vi "SQLite Insert Calibration Value.vi"(7 "Main":string="0", 8 "error in (no error)":errorcluster, 9 "Calibration Value":T1, 11 "VariableName":string) -> (0 "error out":errorcluster)   [LabVIEW 2017, in "SQLite.lvclass"]
doc: "保存校准数据到DB。在保存之前先调用删除原先校准数据模块。\n2015-11-03 15:56:09\n蒋松\njiangsong@outlook.com"
uses:
  SQLite.lvclass
  Calibration Value.ctl
  SQLiteFileName.ctl
  TabelFullName.ctl
  Calibration Kb and Volt.ctl
  Calibration K and b Array.ctl
  Calibration K and b.ctl
  <vilib>/Utility/error.llb/Trim Whitespace.vi
  <userlib>/sushu/sushu.lvlib
  <userlib>/LabSQL/LabSQL.lvlib
panel:
  out "Insert DB String":string
  in  "error in (no error) 2":errorcluster
  in  "OK":bool
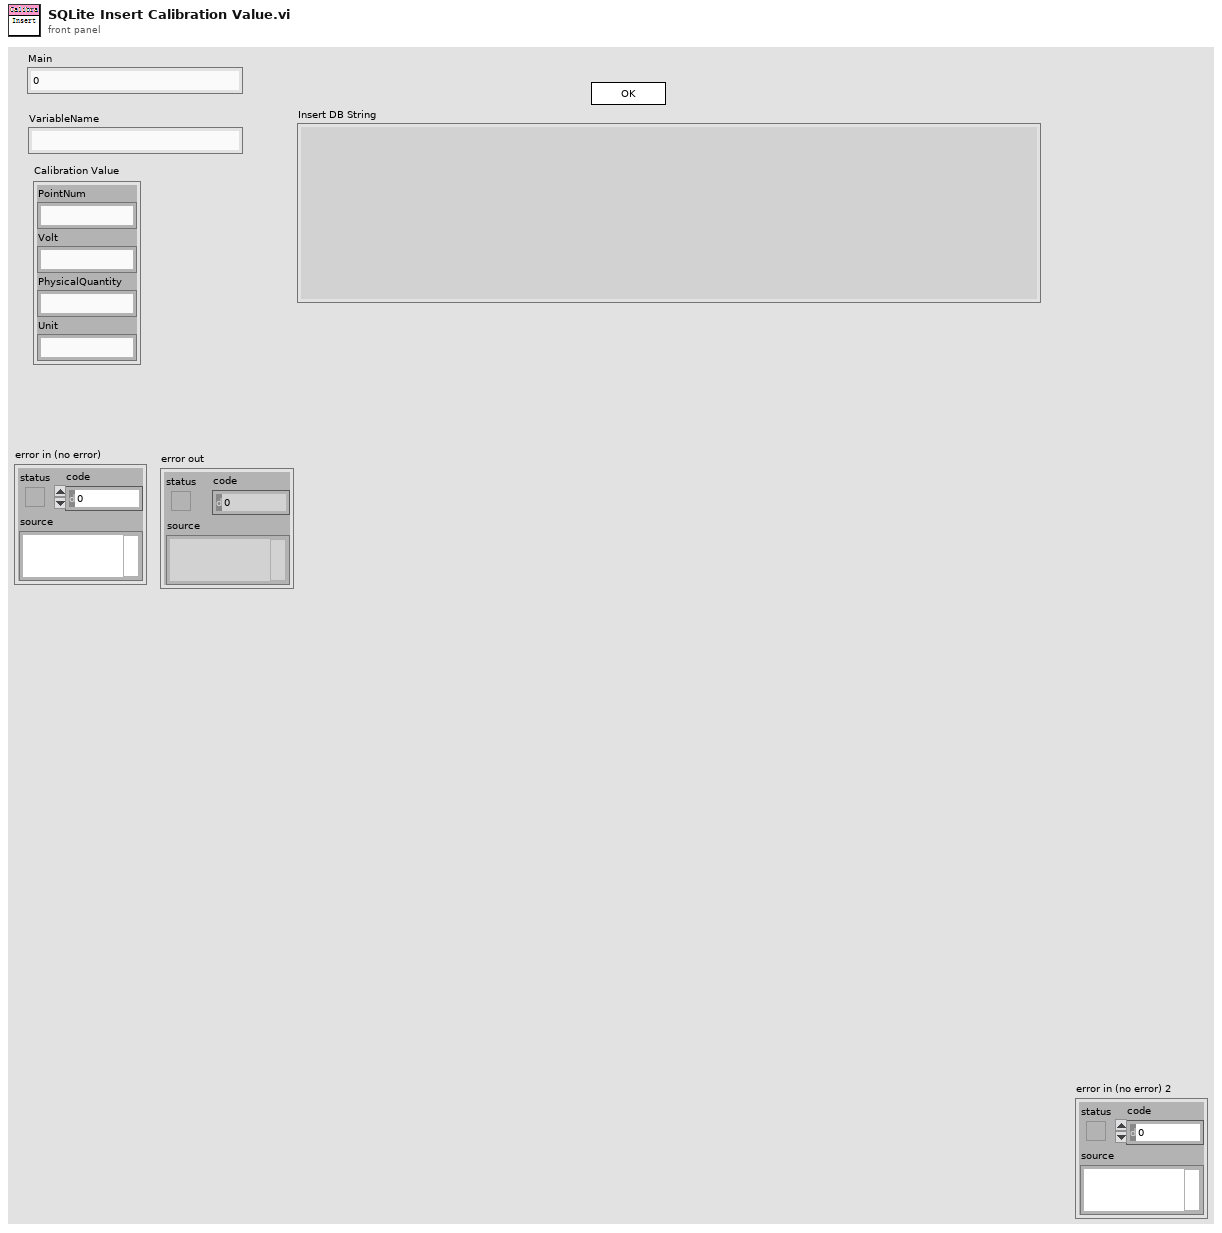
[diagram p1: front panel]
types:
  T1 = typedef "SQLite.lvclass/Calibration Value.ctl" = cluster{"PointNum":string, "Volt":string, "PhysicalQuantity":string, "Unit":string}
  T2 = typedef "SQLite.lvclass/Calibration Kb and Volt.ctl" = cluster{"Kb":T3, "Relation":dbl[][]}
  T3 = typedef "SQLite.lvclass/Calibration K and b Array.ctl" = T4[]
  T4 = typedef "SQLite.lvclass/Calibration K and b.ctl" = cluster{"K":dbl, "b":dbl}
  T5 = typedef "SQLite.lvclass/TabelFullName.ctl" = string
  T6 = typedef "SQLite.lvclass/SQLiteFileName.ctl" = string
  T7 = cluster{"Current VI Reference":refnum<vi>, "Close Panel on Exit?":bool}
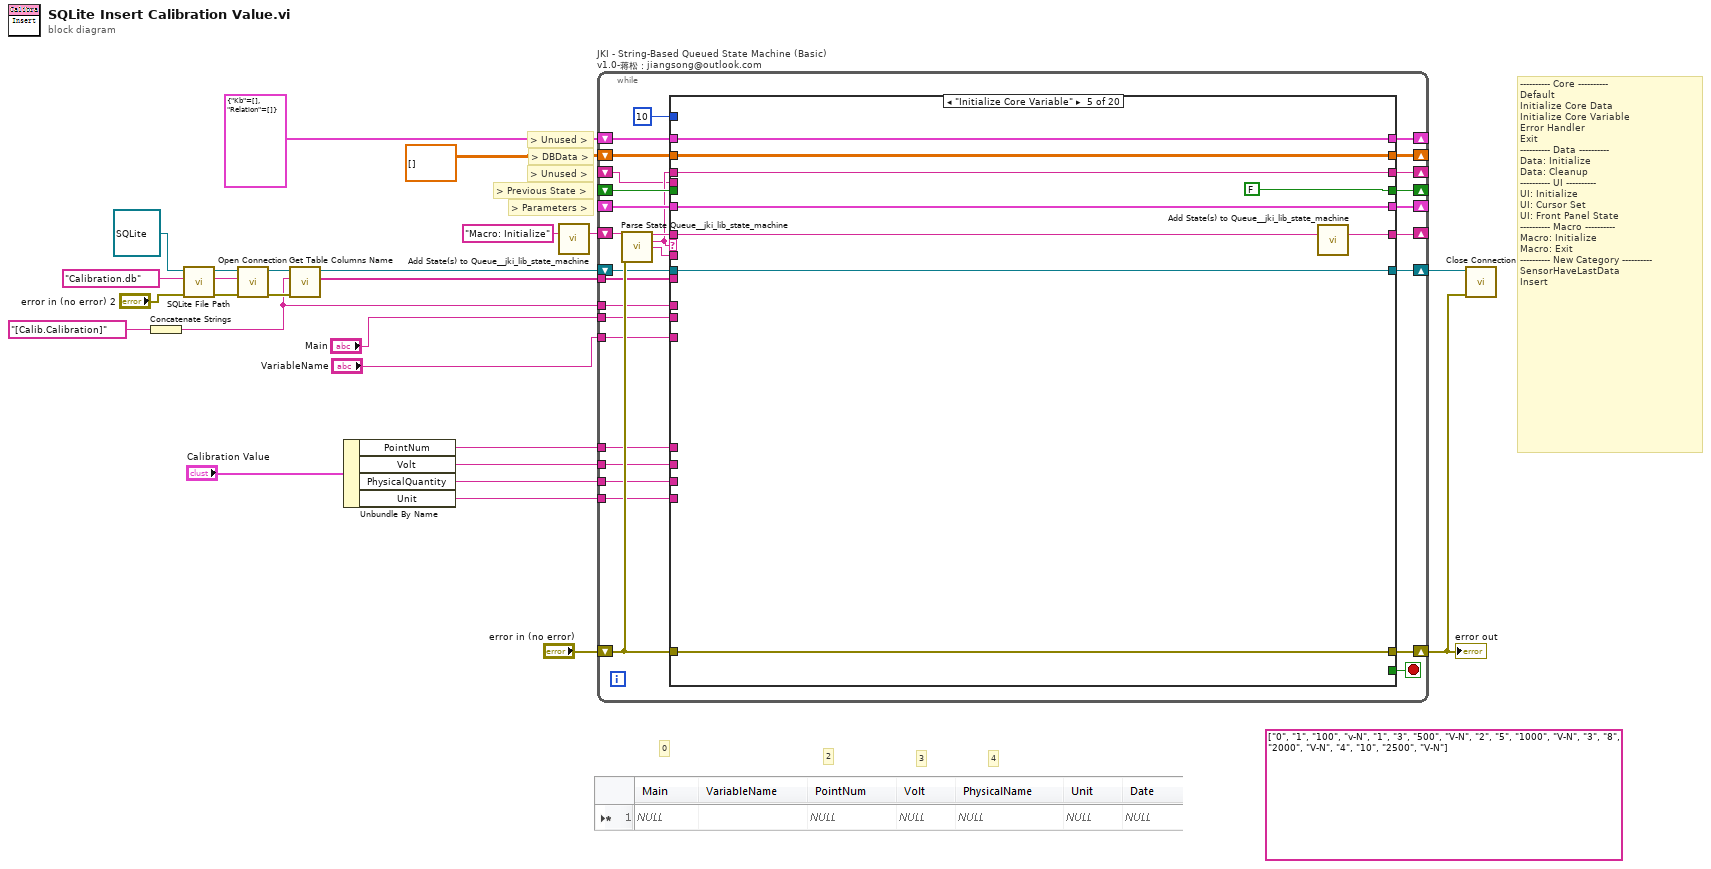
[diagram p0: block diagram]
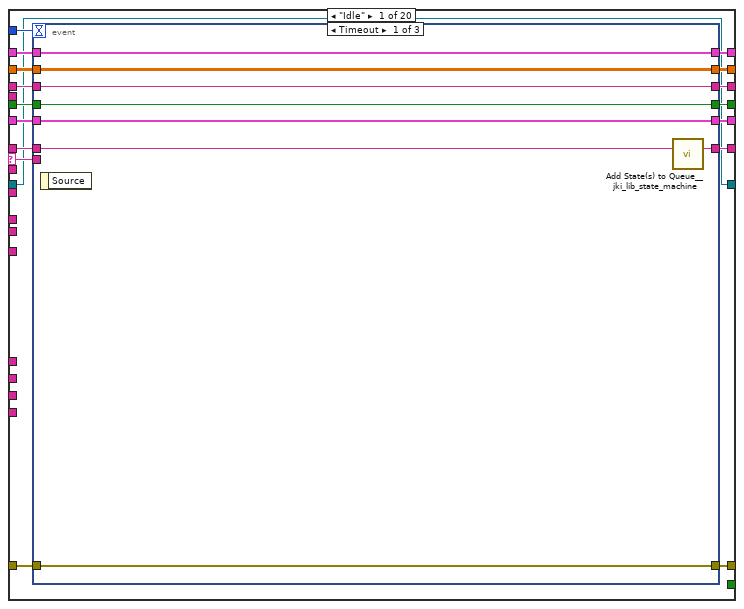
[diagram p2: hidden frame]
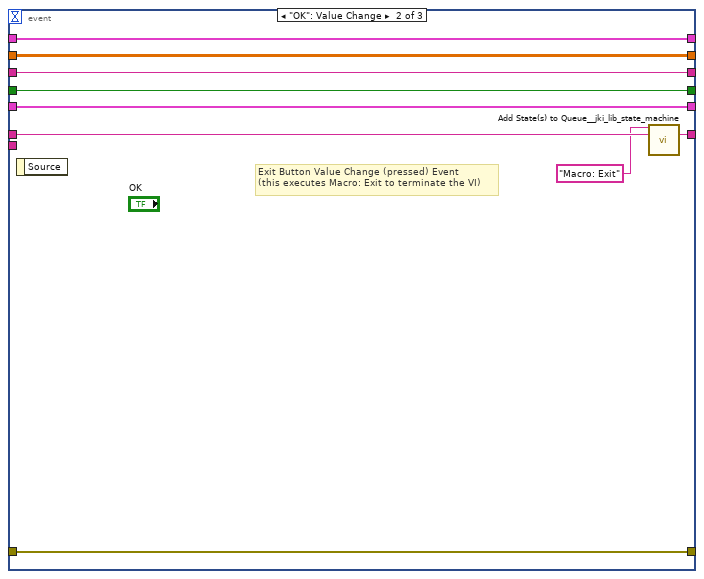
[diagram p3: hidden frame]
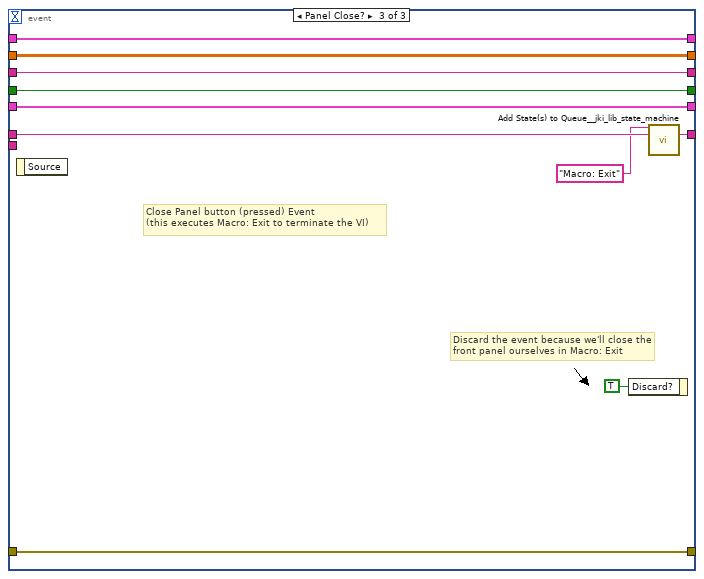
[diagram p4: hidden frame]
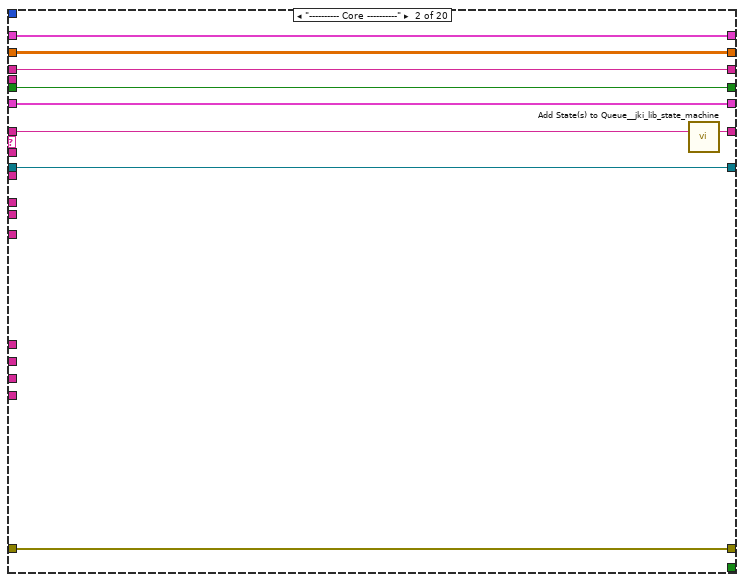
[diagram p5: hidden frame]
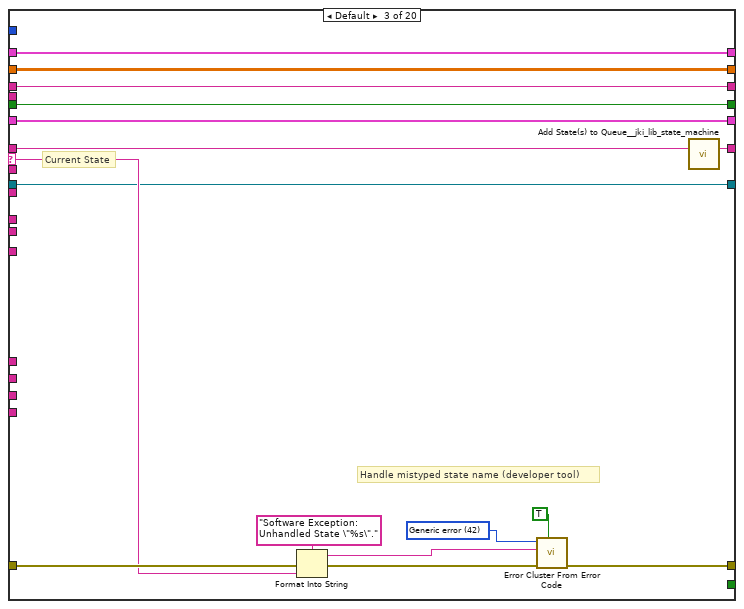
[diagram p6: hidden frame]
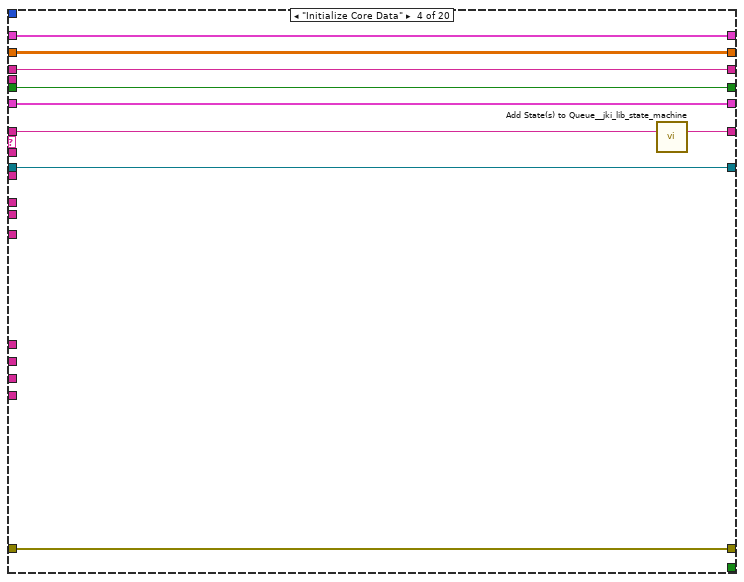
[diagram p7: hidden frame]
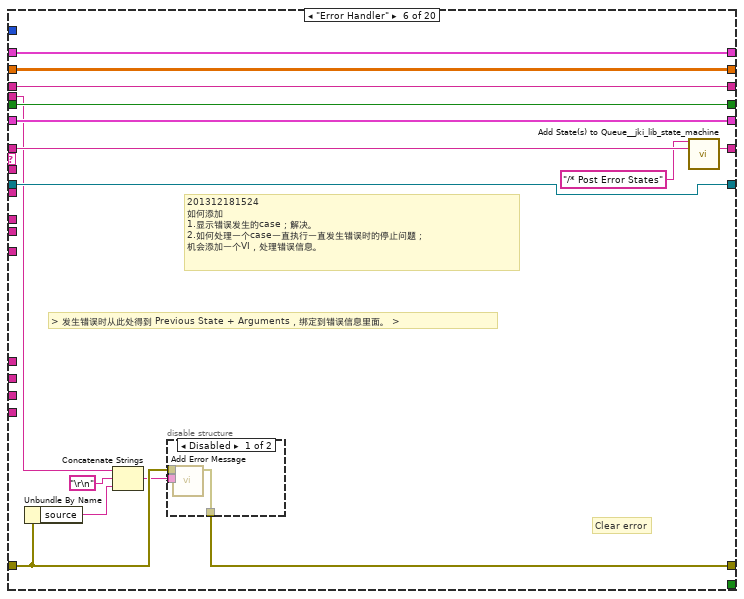
[diagram p8: hidden frame]
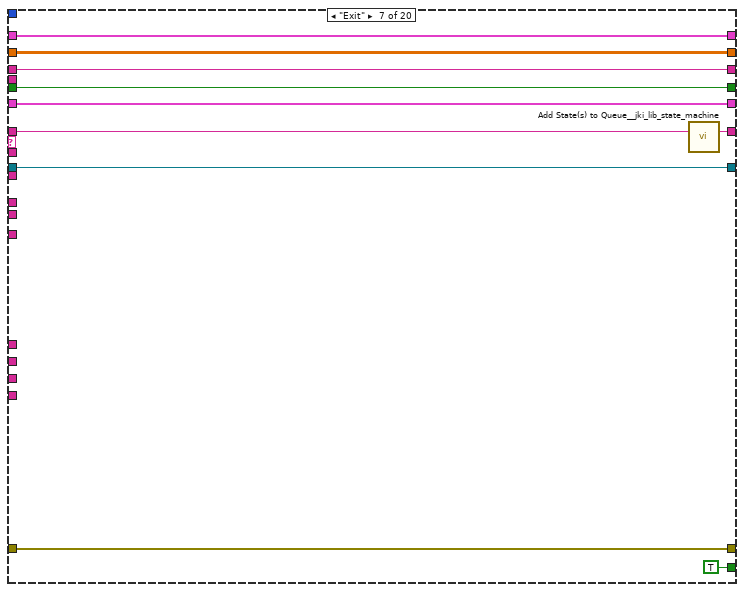
[diagram p10: hidden frame]
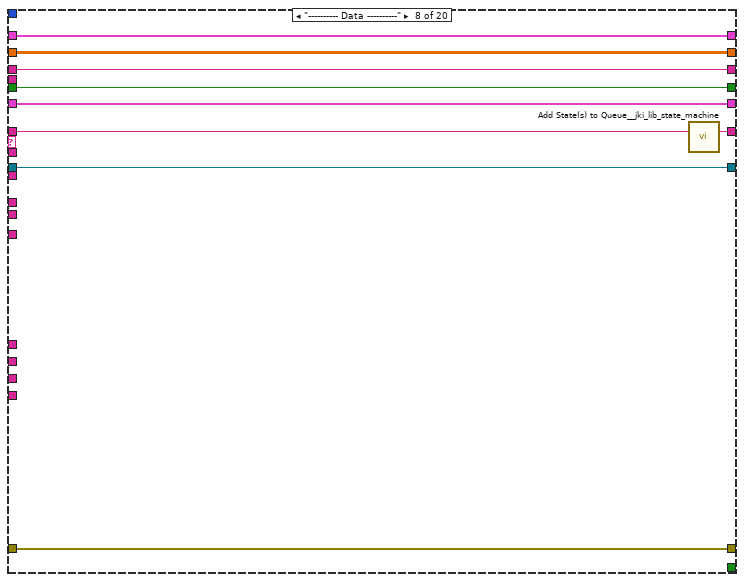
[diagram p11: hidden frame]
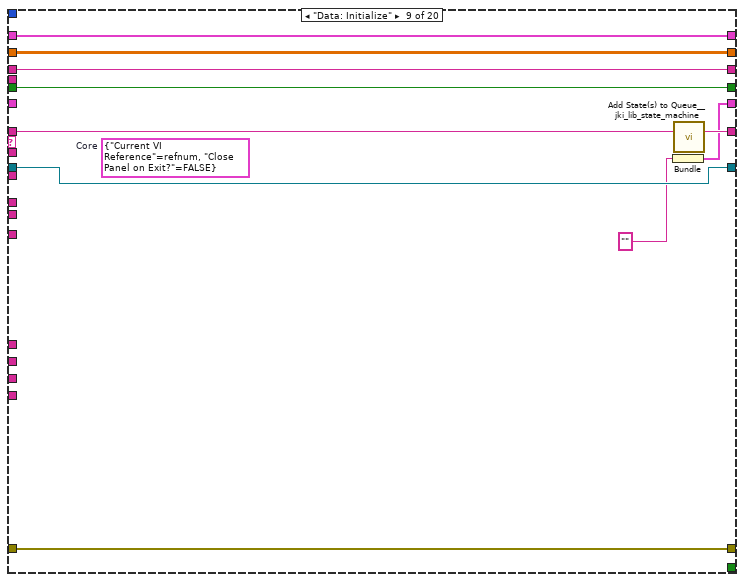
[diagram p12: hidden frame]
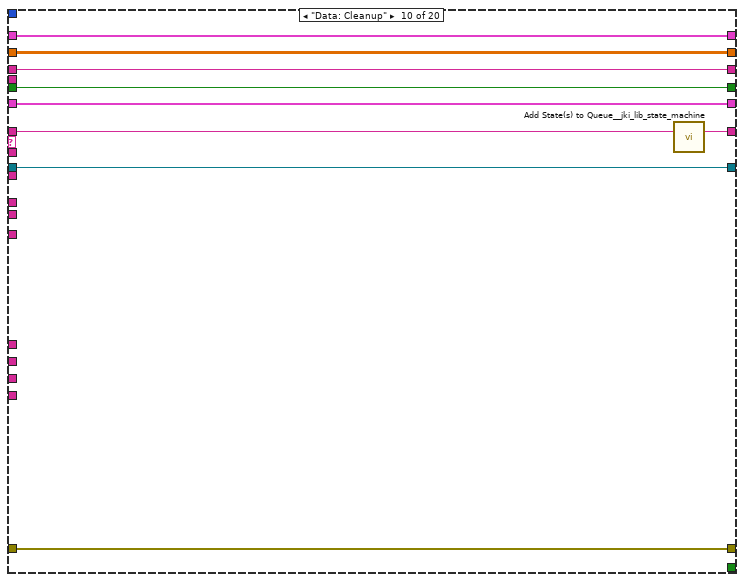
[diagram p13: hidden frame]
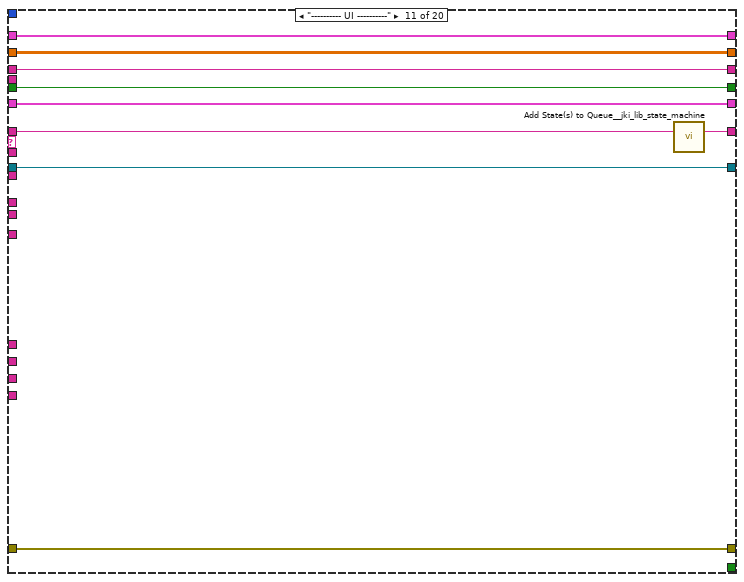
[diagram p14: hidden frame]
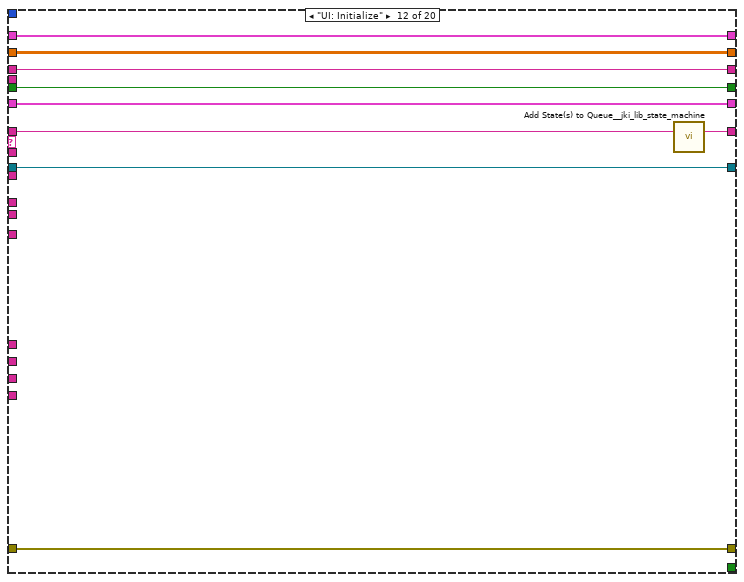
[diagram p15: hidden frame]
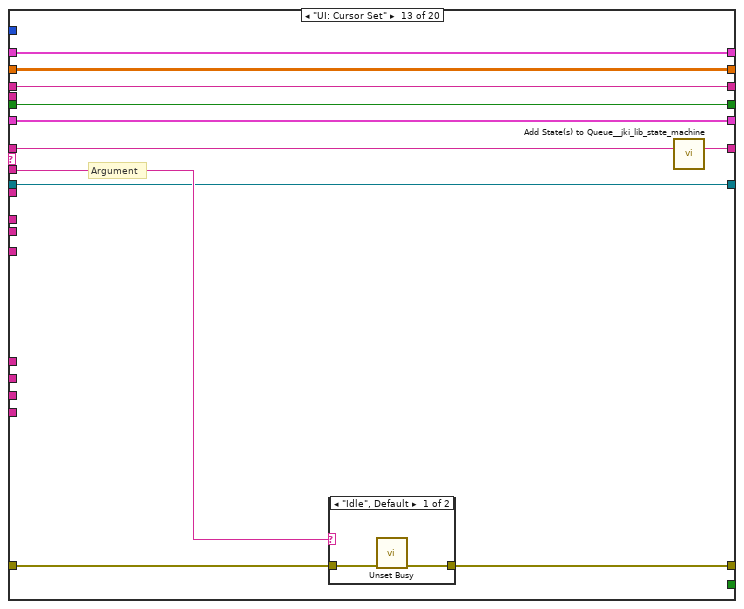
[diagram p16: hidden frame]
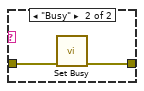
[diagram p17: hidden frame]
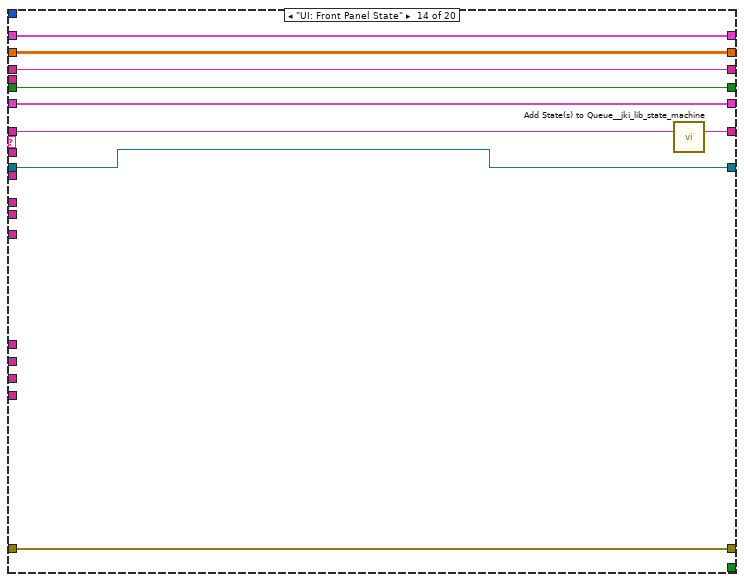
[diagram p18: hidden frame]
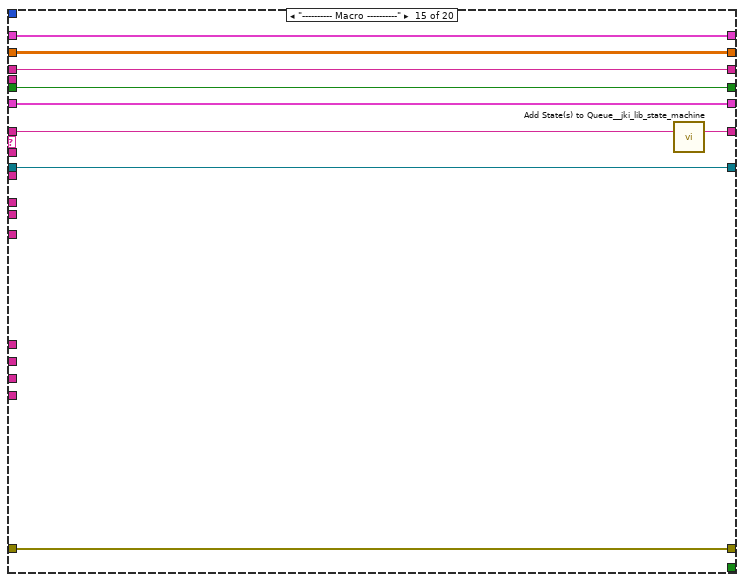
[diagram p19: hidden frame]
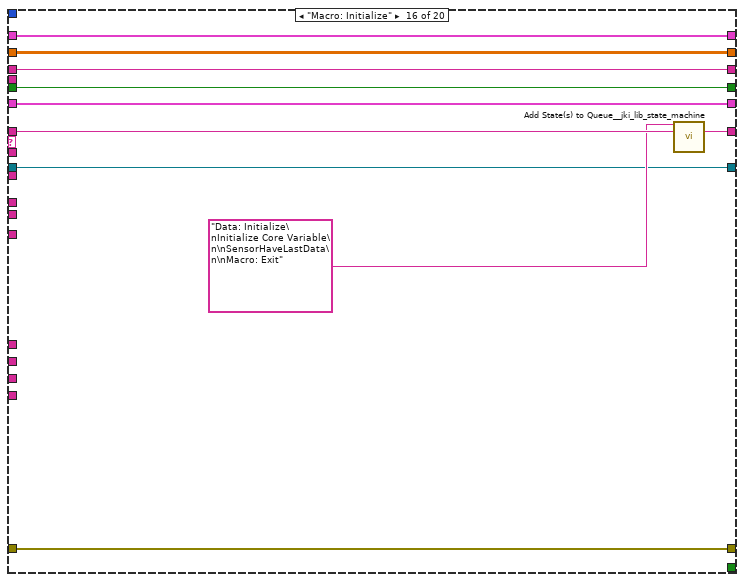
[diagram p20: hidden frame]
diagram:
  (unwired) string[][] [["0", "1", "100", "v-N"], ["1", "3", "500", "V-N"], ["2", "5", "1000", "V-N"], ["3", "8", "2000", "V-N"], ["4", "10", "2500", "V-N"]] ("Result Set 2")
  # "3"
  # "0"
  # "> Parameters >"
  # "> Previous State >"
  # "> Unused >"
  # "> DBData >"
  # "> Unused >"
  # "---------- Core ----------\nDefault\nInitialize Core Data\nInitialize Core Variable\nError Handler\nExit\n---------- Data ----------\nData: Initialize\nData: Cleanup\n---------- UI ----------\nUI: Initialize\nUI: Cursor Set\nUI: Front Panel State\n---------- Macro ----------\nMacro: Initialize\nMacro: Exit\n---------- New Category ----------\nSensorHaveLastData\nInsert"
  # "2"
  # "4"
  n1 = Concatenate Strings(T5 "[Calib.Calibration]" ("TabelFullName")) -> (w9:string)
  n2 = call "SQLite File Path.vi"("error in (no error)"="error in (no error) 2", "SQLiteFileName"=T6 "Calibration.db", "SQLite in"=refnum<class "SQLite.lvclass"> refnum ("SQLite.lvclass")) -> ("error out"=w20:errorcluster, "string"=w15:string, "SQLite out"=w17:refnum<class "SQLite.lvclass">)  [unwired: 6 in]
  n3 = call-dynamic "Open Connection.vi"("error in (no error)"=w20, "ConnectionString"=w15, "HostDB in"=w17) -> ("error out"=w14:errorcluster, "HostDB out"=w13:refnum<class "SQLite.lvclass">)  [unwired: 7 in]
  n4 = call-dynamic "Get Table Columns Name.vi"("error in (no error)"=w14, "TableName"=w9, "HostDB in"=w13) -> ("ColunmsList"=w10:string[], "HostDB out"=w11:refnum<class "SQLite.lvclass">)  [unwired: 4 in, 3 out]
  n5 = Unbundle By Name("Calibration Value") -> ("PointNum"=w4:string, "Volt"=w3:string, "PhysicalQuantity"=w2:string, "Unit"=w1:string)
  n6 = call <vilib>:"Add State(s) to Queue__jki_lib_state_machine.vi"("State(s) in (\"\")"="Macro: Initialize") -> ("States Out"=w26:string)  [unwired: 14 in]
  n7 = while "JKI - String-Based Queued State Machine (Basic) v1.0-蒋松：jiangsong@outlook.com" {
    shift-right: [w53] -> w7
    shift-left: "error in (no error)" -> [w49]
    shift-right: [w52] -> _
    shift-left: w26 -> [w40]
    shift-right: [w45] -> _
    shift-left: dbl[][] [] ("number") -> [w47]
    shift-right: [w46] -> _
    shift-left: T2 {"Kb"=[], "Relation"=[]} ("Calibration") -> [w48]
    shift-right: [w41] -> _
    shift-left: _ -> [w44]
    shift-right: [w42] -> _
    shift-left: _ -> [w33]
    shift-right: [w43] -> _
    shift-left: _ -> [w27]
    tunnel: w10 -> [w39]
    tunnel: w9 -> [w38]
    tunnel: "Main" -> [w37]
    tunnel: "VariableName" -> [w36]
    shift-right: [w34] -> w8
    shift-left: w11 -> [w35]
    tunnel: w4 -> [w32]
    tunnel: w3 -> [w31]
    tunnel: w2 -> [w30]
    tunnel: w1 -> [w29]
    stop <- w51 stop-if-true
    n8 = call <vilib>:"Parse State Queue__jki_lib_state_machine.vi"("State Queue"=w40, "Error In (no error)"=w49) -> ("Remaining States"=w55:string, "Current State"=w28:string, "Arguments"=w54:string)  [unwired: 10 in, 1 out]
    n9 = case shown="\"Initialize Core Variable\"" w28 {
      selector: w28 -> [w58 _ w110 _ _ _ _ _ _ _ _ _ _ _ _ _ _ _ _ _]
      tunnel: w55 -> [w72 w108 w124 w133 w142 w157 w170 w179 w189 w198 w207 w216 w227 w240 w249 w259 w269 w278 w280 w311]
      tunnel: w54 -> [_ _ _ _ _ _ _ _ _ _ _ _ w221 _ _ _ _ _ _ _]
      tunnel: [w70 w106 w111 w128 w140 w144 w163 w173 w184 w190 w201 w210 w219 w232 w243 w253 w264 w273 w288 w312] -> w53
      tunnel: w49 -> [w69 w106 w112 w128 w140 w147 w163 w173 w184 w190 w201 w210 w220 w232 w243 w253 w264 w273 w288 w312]
      tunnel: [w71 w107 w123 w132 w141 w156 w169 w178 w188 w197 w206 w215 w226 w239 w248 w258 w268 w277 w281 w311] -> w52
      tunnel: [_ _ _ _ _ _ TRUE _ _ _ _ _ _ _ _ _ _ _ _ _] -> w51
      tunnel: 10 ("Timeout") -> [w68 _ _ _ _ _ _ _ _ _ _ _ _ _ _ _ _ _ _ _]
      tunnel: w48 -> [w67 w105 w122 w131 w136 w155 w168 w177 w187 w196 w205 w214 w225 w238 w247 w257 w267 w276 w287 w310]
      tunnel: w47 -> [w66 w104 w121 w130 w138 w154 w167 w176 w186 w195 w204 w213 w224 w237 w246 w256 w266 w275 w286 w309]
      tunnel: [w65 w105 w122 w131 w136 w155 w168 w177 w187 w196 w205 w214 w225 w238 w247 w257 w267 w276 w287 w310] -> w46
      tunnel: [w64 w104 w121 w130 w138 w154 w167 w176 w186 w195 w204 w213 w224 w237 w246 w256 w266 w275 w286 w309] -> w45
      tunnel: w28 -> [w62 w103 w120 w129 w134 w153 w166 w175 w185 w194 w203 w212 w223 w236 w245 w255 w265 w274 w285 w308]
      tunnel: w33 -> [w61 w101 w119 w127 _ w150 w162 w172 w182 w192 w200 w209 w218 w234 w242 w251 w262 w271 w284 w307]
      tunnel: w44 -> [w59 w102 w118 w125 w139 w145 w165 w174 _ w193 w202 w211 w222 w235 w244 w254 w263 w272 w283 w306]
      tunnel: [w63 w103 w120 w129 w134 w153 w166 w175 w185 w194 w203 w212 w223 w236 w245 w255 w265 w274 w285 w308] -> w43
      tunnel: [w57 w101 w119 w127 FALSE w150 w162 w172 w182 w192 w200 w209 w218 w234 w242 w251 w262 w271 w284 w307] -> w42
      tunnel: [w60 w102 w118 w125 w139 w145 w165 w174 w183 w193 w202 w211 w222 w235 w244 w254 w263 w272 w283 w306] -> w41
      tunnel: w39 -> [_ _ _ _ _ _ _ _ _ _ _ _ _ _ _ _ _ _ _ w293]
      tunnel: w38 -> [_ _ _ _ _ _ _ _ _ _ _ _ _ _ _ _ _ _ _ w295]
      tunnel: w37 -> [_ _ _ _ _ _ _ _ _ _ _ _ _ _ _ _ _ _ _ w305]
      tunnel: w36 -> [_ _ _ _ _ _ _ _ _ _ _ _ _ _ _ _ _ _ _ w304]
      tunnel: w35 -> [w56 w100 w109 w126 w137 w148 w161 w171 w181 w191 w199 w208 w217 w233 w241 w250 w261 w270 w282 w299]
      tunnel: [w56 w100 w109 w126 w137 w148 w161 w171 w181 w191 w199 w208 w217 w233 w241 w250 w261 w270 w282 w298] -> w34
      tunnel: w32 -> [_ _ _ _ _ _ _ _ _ _ _ _ _ _ _ _ _ _ _ w303]
      tunnel: w31 -> [_ _ _ _ _ _ _ _ _ _ _ _ _ _ _ _ _ _ _ w302]
      tunnel: w30 -> [_ _ _ _ _ _ _ _ _ _ _ _ _ _ _ _ _ _ _ w301]
      tunnel: w29 -> [_ _ _ _ _ _ _ _ _ _ _ _ _ _ _ _ _ _ _ w300]
      tunnel: w27 -> [_ _ _ _ _ w143 _ _ _ _ _ _ _ _ _ _ _ _ _ _]
      frame "Idle" {
        n10 = event shown="[0] Timeout" {
          selector: _ -> [_ _ _]
          dyn-events: _ -> [_ _ _]
          timeout: w68 -> [_ _ _]
          tunnel: w72 -> [w80 w89 w99]
          tunnel: [w79 w88 w98] -> w71
          tunnel: [w78 w87 w97] -> w70
          tunnel: w69 -> [w78 w87 w97]
          tunnel: w67 -> [w77 w86 w96]
          tunnel: w66 -> [w76 w85 w95]
          tunnel: [w77 w86 w96] -> w65
          tunnel: [w76 w85 w95] -> w64
          tunnel: [w75 w84 w94] -> w63
          tunnel: w62 -> [w75 w84 w94]
          tunnel: w61 -> [w73 w81 w90]
          tunnel: [w74 w83 w93] -> w60
          tunnel: w59 -> [w74 w83 w93]
          tunnel: w58 -> [_ _ _]
          tunnel: [w73 w81 w90] -> w57
          event Timeout {
            n11 = event-data() -> ()  [unwired: 1 in, 1 out]
            n12 = call <vilib>:"Add State(s) to Queue__jki_lib_state_machine.vi"("State(s) in (\"\")"=w80) -> ("States Out"=w79:string)  [unwired: 14 in]
          }
          event "OK": Value Change {
            # "Exit Button Value Change (pressed) Event\n(this executes Macro: Exit to terminate the VI)"
            n13 = event-data() -> ()  [unwired: 1 in, 1 out]
            n14 = call <vilib>:"Add State(s) to Queue__jki_lib_state_machine.vi"("State(s) in Front (\"\")"="Macro: Exit", "State(s) in (\"\")"=w89) -> ("States Out"=w88:string)  [unwired: 13 in]
          }
          event Panel Close? {
            # "Discard the event because we'll close the front panel ourselves in Macro: Exit"
            # "Close Panel button (pressed) Event\n(this executes Macro: Exit to terminate the VI)"
            n15 = event-data() -> ()  [unwired: 1 in, 1 out]
            n16 = event-data("Discard?"=TRUE) -> ()  [unwired: 1 in, 1 out]
            n17 = call <vilib>:"Add State(s) to Queue__jki_lib_state_machine.vi"("State(s) in Front (\"\")"="Macro: Exit", "State(s) in (\"\")"=w99) -> ("States Out"=w98:string)  [unwired: 13 in]
          }
        }
      }
      frame "---------- Core ----------" {
        n18 = call <vilib>:"Add State(s) to Queue__jki_lib_state_machine.vi"("State(s) in (\"\")"=w108) -> ("States Out"=w107:string)  [unwired: 14 in]
      }
      frame Default {
        w114 = 42 items=["No error", "Argument error", "Memory is full", "Out of zone", "End of file", "File already open", "Generic file I/O error", "File not found", "File permission error", "Disk is full", "Duplicate path", "Too many files open", "System feature not enabled", "Resource file not found", "Cannot add resource", "Resource not found", "Image not found", "Image memory error", "Pen does not exist", "Config type invalid", "Config token not found", "Config parse error", "Config memory error", "Bad external code format", "Bad external code offset", "External code not present", "Null window", "Destroy window error", "Null menu", "Print aborted", "Bad print record", "Print driver error", "Windows error during printing", "Memory error during printing", "Print dialog error", "Generic print error", "Invalid device refnum", "Device not found", "Device parameter error", "Device unit error", "Cannot open device", "Device call aborted", "Generic error", "Cancelled by user", "Object ID too low", "Object ID too high", "Object not in heap", "Unknown heap", "Unknown object (invalid DefProc)", "Unknown object (DefProc not in table)", "Message out of range", "Invalid (null) method", "Unknown message", "Manager call not supported", "Bad address", "Network operation in progress", "Network operation timed out", "Connection is busy", "Network attribute not supported", "Network error", "Address in use", "System out of memory", "Connection aborted", "Connection refused", "Not connected", "Already connected", "Connection closed", "Initialization error (interapplication manager)", "Bad occurrence", "Wait on unbound occurrence handler", "Occurrence queue overflow", "Datalog type conflict", "Unused", "Unrecognized type (interapplication manager)", "Memory corrupt", "Failed to make temporary DLL", "Old CIN version", "Drag socket not found", "Failed to load drop-object", "Failed to register OLE object", "Failed to release OLE object", "Format specifier type mismatch", "Unknown format specifier", "Too few format specifiers", "Too many format specifiers", "Scan failed", "Newer CIN version", "Error converting to variant", "Runtime menu error", "Password tampered", "Variant attribute not found", "Incompatible variant data type", "Event data is not available", "Event Store is not present", "Occurrence is not found", "Event Queue is not created", "Event info is not available", "Refnum passed is NULL", "Error retrieving Class GUID", "Error retrieving CoClass GUID", "Error retrieving TypeLib GUID.", "Bad built application magic bytes.", "Specific driver is different from the specific driver associated with the Logical Name.", "There is no session opened to the class driver.", "Max Error", "MAX - Error with config objects", "MAX - Error loading configuration", "MAX - Group not supported"]
        # "Current State"
        # "Handle mistyped state name (developer tool)"
        n19 = Format Into String(format string="Software Exception: Unhandled State \"%s\"." ("message"), error in=w112, w110) -> (resulting string=w115:string, error out=w116:errorcluster)  [unwired: 1 in]
        n20 = call <vilib>:"Error Cluster From Error Code.vi"("show call chain? (False)"=TRUE, "error in (no error)"=w116, "error message (\"\")"=w115, "error code (0)"=w114) -> ("error out"=w111:errorcluster)  [unwired: 5 in]
        n21 = call <vilib>:"Add State(s) to Queue__jki_lib_state_machine.vi"("State(s) in (\"\")"=w124) -> ("States Out"=w123:string)  [unwired: 14 in]
      }
      frame "Initialize Core Data" {
        n22 = call <vilib>:"Add State(s) to Queue__jki_lib_state_machine.vi"("State(s) in (\"\")"=w133) -> ("States Out"=w132:string)  [unwired: 14 in]
      }
      frame "Initialize Core Variable" {
        n23 = call <vilib>:"Add State(s) to Queue__jki_lib_state_machine.vi"("State(s) in (\"\")"=w142) -> ("States Out"=w141:string)  [unwired: 14 in]
      }
      frame "Error Handler" {
        # "> 发生错误时从此处得到 Previous State + Arguments，绑定到错误信息里面。 >"
        # "201312181524\n如何添加\n1.显示错误发生的case；解决。\n2.如何处理一个case一直执行一直发生错误时的停止问题；\n机会添加一个VI，处理错误信息。"
        # "Clear error"
        n24 = Unbundle By Name(w147) -> ("source"=w149:string)
        n25 = Concatenate Strings(w143, "\r\n", w149) -> (w146:string)
        n26 = disable-structure shown="Disabled" {
          disable-tunnel: w147 -> [w160 _]
          disable-tunnel: w146 -> [w159 _]
          disable-tunnel: [w158 _] -> w144
          frame Disabled {
            n27 = call <userlib>:"Add Error Message.vi"("ErrorMessages"=w159, "error in (no error)"=w160) -> ("error out"=w158:errorcluster)  [unwired: 9 in]
          }
          frame Enabled {
          }
        }
        n28 = call <vilib>:"Add State(s) to Queue__jki_lib_state_machine.vi"("State(s) in Front (\"\")"="/* Post Error States", "State(s) in (\"\")"=w157) -> ("States Out"=w156:string)  [unwired: 13 in]
      }
      frame "Exit" {
        n29 = call <vilib>:"Add State(s) to Queue__jki_lib_state_machine.vi"("State(s) in (\"\")"=w170) -> ("States Out"=w169:string)  [unwired: 14 in]
      }
      frame "---------- Data ----------" {
        n30 = call <vilib>:"Add State(s) to Queue__jki_lib_state_machine.vi"("State(s) in (\"\")"=w179) -> ("States Out"=w178:string)  [unwired: 14 in]
      }
      frame "Data: Initialize" {
        (unwired) T7 {"Current VI Reference"=refnum, "Close Panel on Exit?"=FALSE}  # Core
        n31 = Bundle("") -> (w183:cluster{string})  [unwired: 1 in]
        n32 = call <vilib>:"Add State(s) to Queue__jki_lib_state_machine.vi"("State(s) in (\"\")"=w189) -> ("States Out"=w188:string)  [unwired: 14 in]
      }
      frame "Data: Cleanup" {
        n33 = call <vilib>:"Add State(s) to Queue__jki_lib_state_machine.vi"("State(s) in (\"\")"=w198) -> ("States Out"=w197:string)  [unwired: 14 in]
      }
      frame "---------- UI ----------" {
        n34 = call <vilib>:"Add State(s) to Queue__jki_lib_state_machine.vi"("State(s) in (\"\")"=w207) -> ("States Out"=w206:string)  [unwired: 14 in]
      }
      frame "UI: Initialize" {
        n35 = call <vilib>:"Add State(s) to Queue__jki_lib_state_machine.vi"("State(s) in (\"\")"=w216) -> ("States Out"=w215:string)  [unwired: 14 in]
      }
      frame "UI: Cursor Set" {
        # "Argument"
        n36 = case shown="\"Idle\", Default" w221 {
          tunnel: w220 -> [w229 w231]
          tunnel: [w228 w230] -> w219
          frame "Idle", Default {
            n37 = call <vilib>:"Unset Busy.vi"("error in (no error)"=w229) -> ("error out"=w228:errorcluster)  [unwired: 10 in]
          }
          frame "Busy" {
            n38 = call <vilib>:"Set Busy.vi"("error in (no error)"=w231) -> ("error out"=w230:errorcluster)  [unwired: 9 in, 1 out]
          }
        }
        n39 = call <vilib>:"Add State(s) to Queue__jki_lib_state_machine.vi"("State(s) in (\"\")"=w227) -> ("States Out"=w226:string)  [unwired: 14 in]
      }
      frame "UI: Front Panel State" {
        n40 = call <vilib>:"Add State(s) to Queue__jki_lib_state_machine.vi"("State(s) in (\"\")"=w240) -> ("States Out"=w239:string)  [unwired: 14 in]
      }
      frame "---------- Macro ----------" {
        n41 = call <vilib>:"Add State(s) to Queue__jki_lib_state_machine.vi"("State(s) in (\"\")"=w249) -> ("States Out"=w248:string)  [unwired: 14 in]
      }
      frame "Macro: Initialize" {
        n42 = call <vilib>:"Add State(s) to Queue__jki_lib_state_machine.vi"("State(s) in Front (\"\")"="Data: Initialize\nInitialize Core Variable\n\nSensorHaveLastData\n\nMacro: Exit", "State(s) in (\"\")"=w259) -> ("States Out"=w258:string)  [unwired: 13 in]
      }
      frame "Macro: Exit" {
        n43 = call <vilib>:"Add State(s) to Queue__jki_lib_state_machine.vi"("State(s) in Front (\"\")"="Data: Cleanup\nExit", "State(s) in (\"\")"=w269) -> ("States Out"=w268:string)  [unwired: 13 in]
      }
      frame "---------- New Category ----------" {
        n44 = call <vilib>:"Add State(s) to Queue__jki_lib_state_machine.vi"("State(s) in (\"\")"=w278) -> ("States Out"=w277:string)  [unwired: 14 in]
      }
      frame "SensorHaveLastData" {
        n45 = call <vilib>:"Add State(s) to Queue__jki_lib_state_machine.vi"("State(s) in Front (\"\")"="Insert" ("State(s) in Front (\"\")"), "State(s) in (\"\")"=w280) -> ("States Out"=w281:string)  [unwired: 13 in]
      }
      frame "Insert" {
        n46 = Build Array(w305, w304, w303, w302, w301, w300) -> (w290:string[])
        n47 = Array Subset(array=w293, index=0, length=6) -> (w294:string[])
        n48 = call <userlib>:"SQL_Insert DB Table.vi"("DB Type"=enum16{"Other", "SQL2008", "SQLite"}."SQLite", "ColumnsValue"=w290, "ColumnsName"=w294, "Table Name"=w295) -> ("Insert DB String"=w296:string)  [unwired: 7 in]
        "Insert DB String" <- w296
        n49 = call-dynamic "SQL Execute.vi"("Return Data (T)"=FALSE, "Command Text"=w296, "HostDB in"=w299) -> ("HostDB out"=w298:refnum<class "SQLite.lvclass">)  [unwired: 4 in, 4 out]
      }
    }
  }
  "error out" <- w7
  n50 = call-dynamic "Close Connection.vi"("error in (no error)"=w7, "HostDB in"=w8) -> ()  [unwired: 8 in, 2 out]
